vi "joe_johnson_state_setpoints.vi"(11 "joe_johnson_state":T1=enum."down") -> (3 "setpoint":dbl)   [LabVIEW 2011]
uses:
  joe_johnson_state.ctl
panel:
  in  "Joe Johnson States":dbl[](array[numeric])=[1.1, -0.15, 0.82, 0.42, 0.63, 0.42, 0.42]
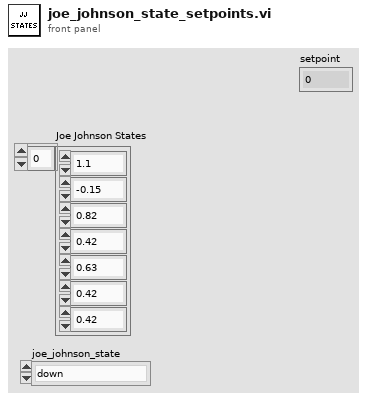
[diagram p1: front panel]
types:
  T1 = typedef "joe_johnson_state.ctl" = enum16{"fold", "down", "up", "ramp", "bridge_lift", "manual", "ramp_stay"}
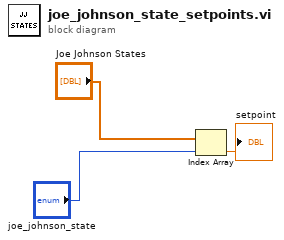
[diagram p0: block diagram]
diagram:
  n1 = Index Array(array="Joe Johnson States", index="joe_johnson_state") -> (element=→"setpoint":dbl)
